vi "Generate Snake.vi"(11 "Length":u32) -> (3 "Snake":u32[](array[colorbox]))   [LabVIEW 2025]
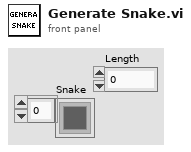
[diagram p1: front panel]
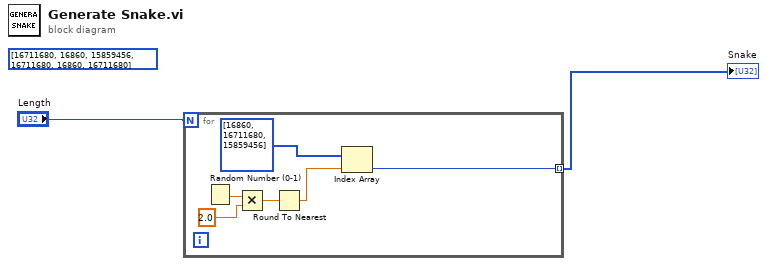
[diagram p0: block diagram]
diagram:
  (unwired) u32[] [16711680, 16860, 15859456, 16711680, 16860, 16711680] ("Snake")
  n1 = for {
    N: "Length" -> [_]
    tunnel: [w4] -> w1 mode=indexing
    n2 = Random Number (0-1)() -> (number: 0 to 1=w7:dbl)
    n3 = Multiply(x=w7, y=2.0) -> (x*y=w5:dbl)
    n4 = Round To Nearest(number=w5) -> (nearest integer value=w3:dbl)
    n5 = Index Array(array=u32[] [16860, 16711680, 15859456], index=w3) -> (element=w4:u32)
  }
  "Snake" <- w1
